vi "Config-BaudRate.vi"(8 "error in (no error)":errorcluster, 10 "Def-PreConfig-BaudRate":T1={"Channel Num"=0, "BaudRate"=125000} {"BaudRate" items=["1 MBaud"=1000000, "800 KBaud"=800000, "500 KBaud"=500000, "400 KBaud"=400000, "250 KBaud"=250000, "200 KBaud"=200000, "160 KBaud"=160000, "125 KBaud"=125000, "100 KBaud"=100000, "83.3 KBaud"=83333, "80 KBaud"=80000, "62.5 KBaud"=62500, "50 KBaud"=50000, "40 KBaud"=40000, "33.3 KBaud"=33333, "<Custom>"=0]}, 11 "Class-Interface in":refnum<class "Class-Interface.lvclass">) -> (0 "error out":errorcluster, 3 "Class-Interface out":refnum<class "Class-Interface.lvclass">)   [LabVIEW 2019, in "CAN-Interface.lvlib" / "Class-Interface.lvclass"]
uses:
  Class-Interface.lvclass
  TypeDef/Def-Config-BaudRate.ctl
  TypeDef/Def-BaudRate.ctl
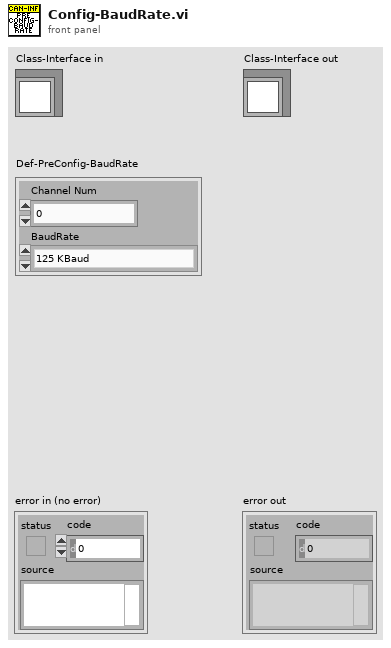
[diagram p1: front panel]
types:
  T1 = typedef "CAN-Interface.lvlib/Class-Interface.lvclass/Def-Config-BaudRate.ctl" = cluster{"Channel Num":u32, "BaudRate":T2}
  T2 = typedef "CAN-Interface.lvlib/Class-Interface.lvclass/Def-BaudRate.ctl" = u32
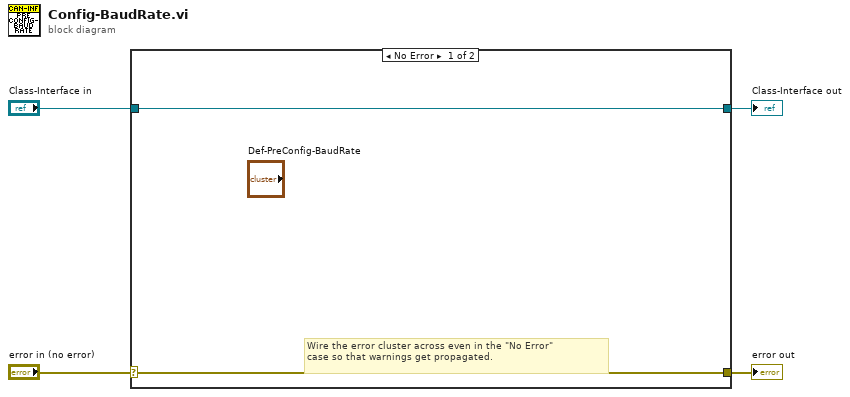
[diagram p0: block diagram]
diagram:
  n1 = case shown="No Error" "error in (no error)" {
    selector: "error in (no error)" -> [w5 w8]
    tunnel: [w5 w8] -> w3
    tunnel: [w6 w7] -> w1
    tunnel: "Class-Interface in" -> [w6 w7]
    frame No Error {
      # "Wire the error cluster across even in the \"No Error\"\ncase so that warnings get propagated."
    }
    frame Error {
    }
  }
  "error out" <- w3
  "Class-Interface out" <- w1
